vi "DAQNavi Read (Analog 2D U16 NChan NSamp).vi"(8 "error in (no error)":errorcluster, 9 "number of samples per channel to read":u32=1000, 10 "timeout":dbl=10.0 format="%0.2f", 11 "task in":i32) -> (0 "error out":errorcluster, 1 "markBuf":cluster{"Data Index":i64, "Src Id":i64}[](array[cluster]), 2 "data":u16[][](array[numeric]), 3 "task out":i32)   [LabVIEW 2020]
uses:
  DAQNavi_LV.dll
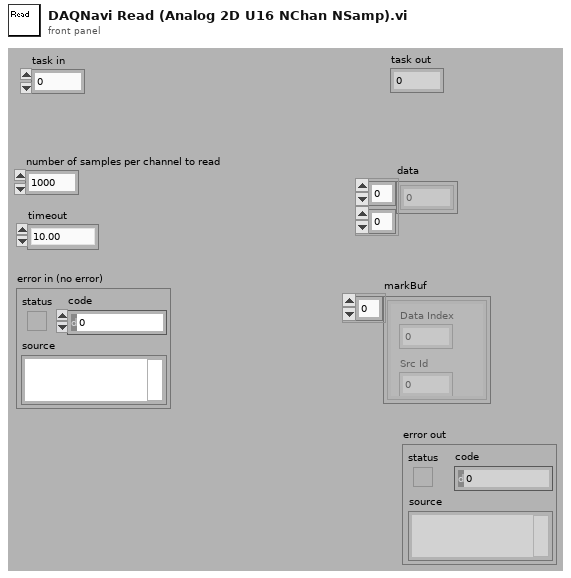
[diagram p1: front panel]
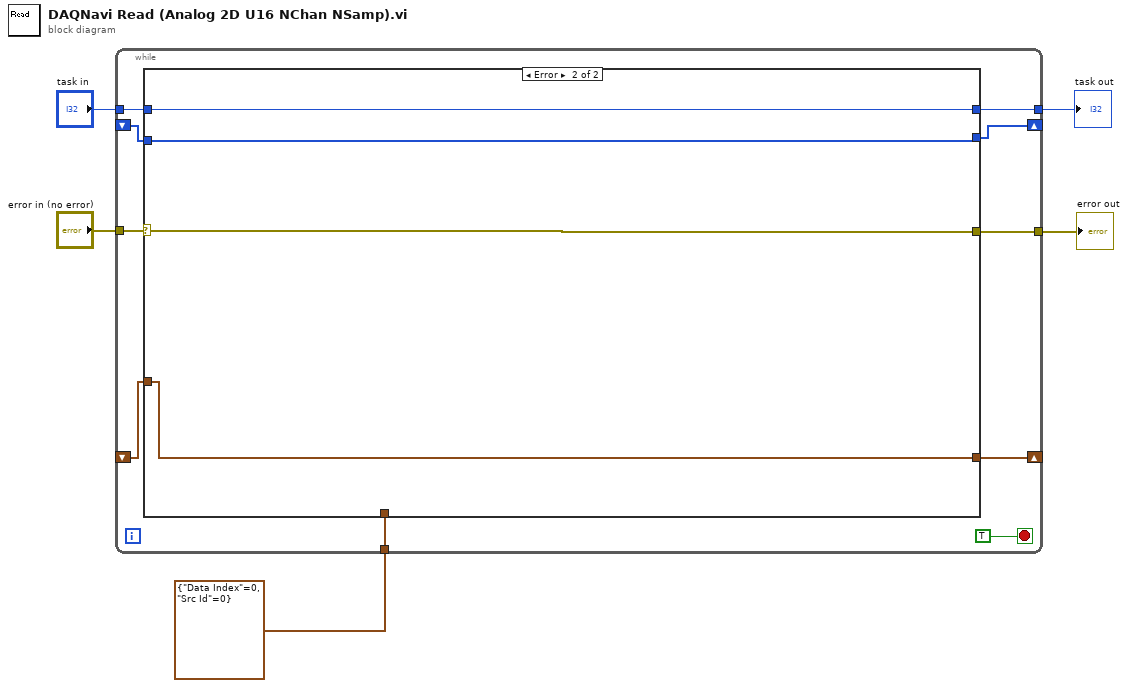
[diagram p0: block diagram]
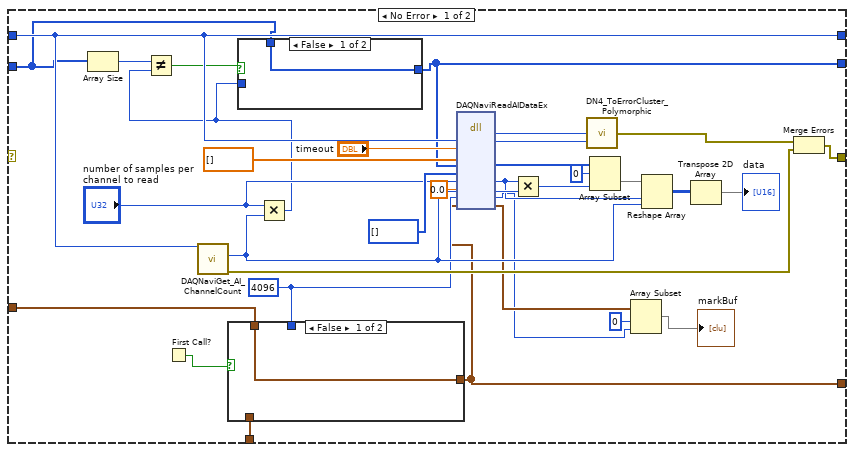
[diagram p2: hidden frame]
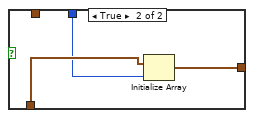
[diagram p3: hidden frame]
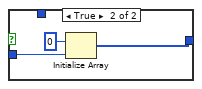
[diagram p4: hidden frame]
diagram:
  n1 = while {
    tunnel: "task in" -> [w15]
    tunnel: "error in (no error)" -> [w14]
    tunnel: [w13] -> w3
    tunnel: [w12] -> w2
    shift-right: [w9] -> _
    shift-left: _ -> [w10]
    tunnel: cluster{"Data Index":i64, "Src Id":i64} {"Data Index"=0, "Src Id"=0} -> [w8]
    shift-right: [w7] -> _
    shift-left: _ -> [w6]
    stop <- TRUE stop-if-true
    n2 = case shown="Error" w14 {
      selector: w14 -> [_ w59]
      tunnel: w15 -> [w42 w60]
      tunnel: [w42 w60] -> w13
      tunnel: [w39 w59] -> w12
      tunnel: w10 -> [w27 w57]
      tunnel: [w26 w57] -> w9
      tunnel: w8 -> [w23 _]
      tunnel: [w21 w58] -> w7
      tunnel: w6 -> [w20 w58]
      frame No Error {
        w22 = 4096
        n3 = Array Size(array=w27) -> (size(s)=w30:i32)
        n4 = First Call?() -> (First Call?: T/F=w24:bool)
        n5 = call "DAQNaviGet_AI_ChannelCount.vi"("task in"=w42) -> ("error out"=w40:errorcluster, "channel count"=w35:i32)  [unwired: 1 in, 8 out]
        n6 = case shown="False" w24 {
          tunnel: w23 -> [_ w52]
          tunnel: w22 -> [_ w51]
          tunnel: [w49 w50] -> w21
          tunnel: w20 -> [w49 _]
          frame False {
          }
          frame True {
            n7 = Initialize Array(w52, w51) -> (w50:cluster{"Data Index":i64, "Src Id":i64}[])
          }
        }
        n8 = Multiply(x="number of samples per channel to read", y=w35) -> (x*y=w28:u32)
        n9 = Not Equal?(x=w30, y=w28) -> (x != y?=w29:bool)
        n10 = case shown="False" w29 {
          tunnel: [w53 w55] -> w26
          tunnel: w28 -> [_ w54]
          tunnel: w27 -> [w53 _]
          frame False {
          }
          frame True {
            n11 = Initialize Array(u16 0 ("element"), w54) -> (w55:u16[])
          }
        }
        n12 = dll-call lib="DAQNavi_LV.dll" fn="DAQNaviReadAIDataEx"("taskID"=w42, "timeout"="timeout", "scaledData"=dbl[] [], "rawData16"=w26, "rawData32"=u32[] [], "samples"="number of samples per channel to read", "startTime"=0.0, "markCount"=w22, "markBuf"=w21) -> ("return type"=w45:i32, "taskID"=w31:i32, "rawData16"=w44:u16[], "samples"=w33:u32, "markCount"=w17:i32, "markBuf"=w19:cluster{"Data Index":i64, "Src Id":i64}[])  [unwired: 4 in, 5 out]
        n13 = Multiply(x=w33, y=w35) -> (x*y=w34:u32)
        n14 = call "DN4_ToErrorCluster_Polymorphic.vi"("task id"=w31, "error code"=w45) -> ("error out"=w41:errorcluster)  [unwired: 3 out]
        n15 = Array Subset(array=w44, index=0, length=w34) -> (w38:u16[])
        n16 = Array Subset(array=w19, index=0, length=w17) -> (→"markBuf":cluster{"Data Index":i64, "Src Id":i64}[])
        n17 = Reshape Array(w38, w33, w35) -> (w37:u16[][])
        n18 = Transpose 2D Array(2D array=w37) -> (transposed array=→"data":u16[][])
        n19 = Merge Errors(w41, w40) -> (w39:errorcluster)
      }
      frame Error {
      }
    }
  }
  "task out" <- w3
  "error out" <- w2
